vi "objects-hidden-by-structures.vi"() -> ()   [LabVIEW 2025]
panel:
  out "Numeric":i32
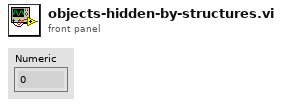
[diagram p1: front panel]
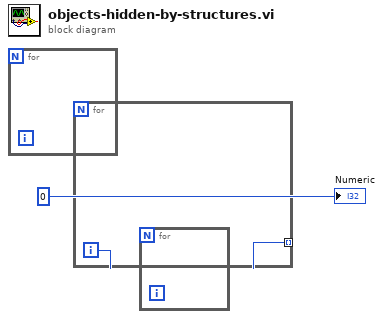
[diagram p0: block diagram]
diagram:
  n1 = for {
  }
  n2 = for {
    tunnel: [w2] -> _ mode=indexing
    i -> [w2]
    n3 = for {
    }
  }
  "Numeric" <- 0
